vi "Failure Message.vi"() -> ()   [LabVIEW 2017, in "Assertions.Tests.lvlib" / "Assert String Starts With.lvlib"]
uses:
  Assert String Starts With.lvlib
  src/Transparent Assertions/Assertions/Assertions.lvlib
panel:
  out "error out":errorcluster
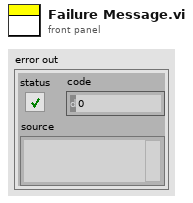
[diagram p1: front panel]
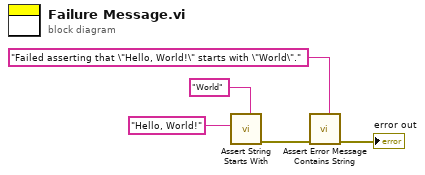
[diagram p0: block diagram]
diagram:
  n1 = call "Assert String Starts With.vi"("Prefix"="World", "String"="Hello, World!") -> ("error out"=w3:errorcluster)  [unwired: 9 in]
  n2 = call "Assert Error Message Contains String.vi"("Expected"="Failed asserting that \"Hello, World!\" starts with \"World\".", "error in (no error)"=w3) -> ("error out"=→"error out":errorcluster)  [unwired: 9 in]
